vi "UHR-Fleezers Control (host) -Leonardo 04-2018 V4_fish.vi"(0 "Tab Green FB":T5(tab)=enum."Trap Control (RF)") -> ()   [LabVIEW 2014] (continued)
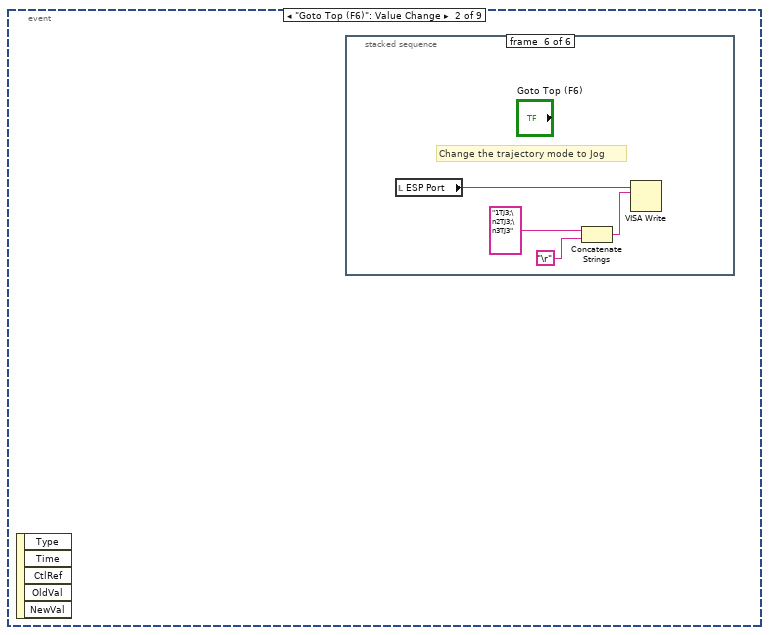
[diagram p4: hidden frame]
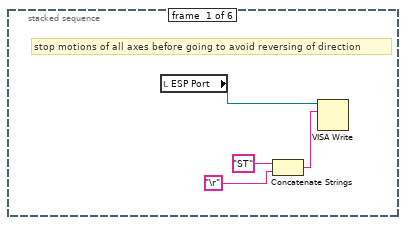
[diagram p5: hidden frame]
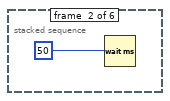
[diagram p6: hidden frame]
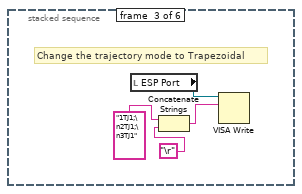
[diagram p7: hidden frame]
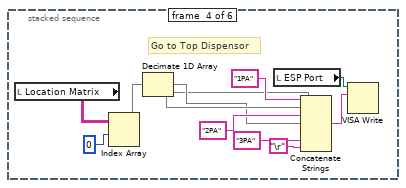
[diagram p8: hidden frame]
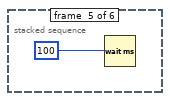
[diagram p9: hidden frame]
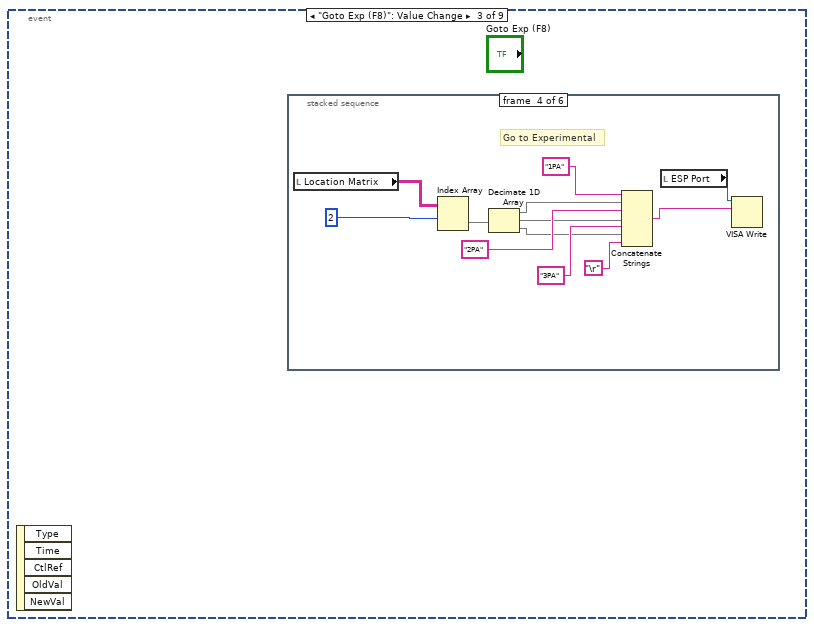
[diagram p10: hidden frame]
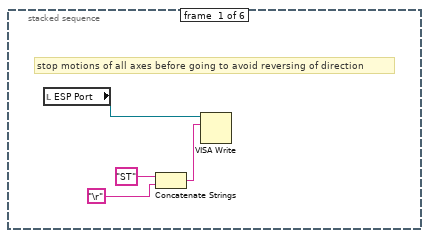
[diagram p11: hidden frame]
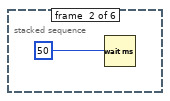
[diagram p12: hidden frame]
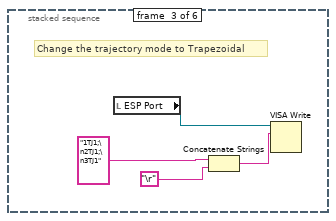
[diagram p13: hidden frame]
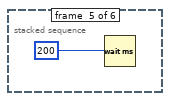
[diagram p14: hidden frame]
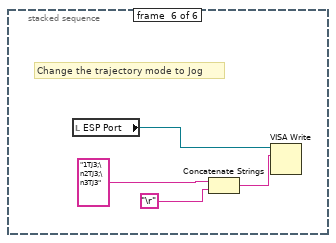
[diagram p15: hidden frame]
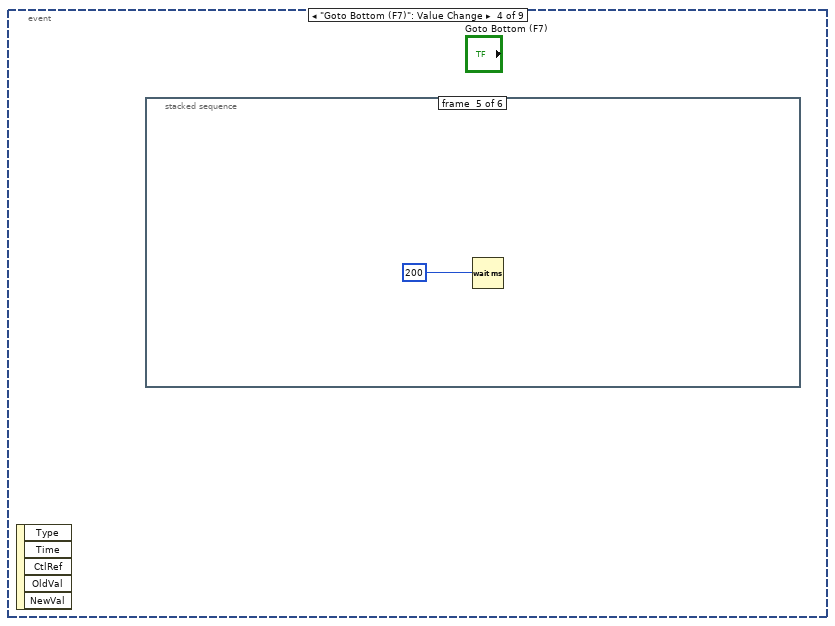
[diagram p16: hidden frame]
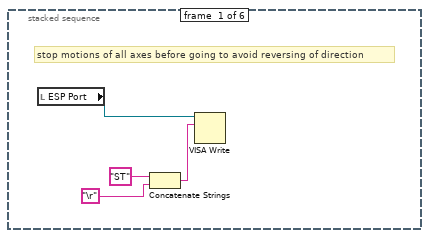
[diagram p17: hidden frame]
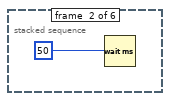
[diagram p18: hidden frame]
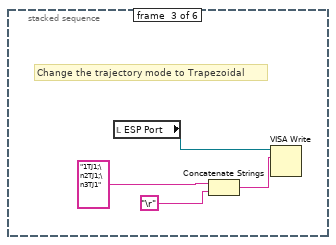
[diagram p19: hidden frame]
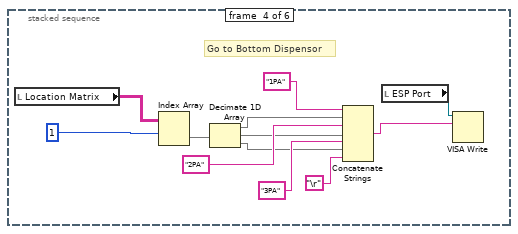
[diagram p20: hidden frame]
          tunnel: w3897 -> [_ w3916]
          tunnel: w3896 -> [_ w3915]
          tunnel: w3895 -> [_ w3913]
          tunnel: w3894 -> [_ w3911]
          tunnel: w3893 -> [_ w3910]
          tunnel: w3892 -> [_ w3909]
          tunnel: w3891 -> [_ w3908]
          tunnel: w3890 -> [_ w3907]
          tunnel: w3889 -> [_ w3906]
          tunnel: w3888 -> [_ w3905]
          frame False {
          }
          frame True {
            n2343 = Multiply(x=w3914, y=w3913) -> (x*y=→"Time (s)":dbl)
            n2344 = Less Or Equal?(x=w3914, y=w3922) -> (x <= y?=w3926:bool)
            n2345 = Or(x="Stop Saving", y="Abort save 2") -> (x .or. y?=w3918:bool)
            n2346 = Not(x=w3918) -> (.not. x?=w3927:bool)
            n2347 = And(x=w3926, y=w3927) -> (x .and. y?=w3925:bool)
            n2348 = case shown="True" w3925 {
              tunnel: w3928 -> [w3935 w4003]
              tunnel: [0.0 w4006] -> w3921
              tunnel: w3914 -> [_ w4004]
              tunnel: w3922 -> [_ w4005]
              tunnel: w3924 -> [_ w4000]
              tunnel: w3923 -> [_ _]
              tunnel: w3917 -> [w3933 w3993]
              tunnel: w3916 -> [w3932 w3994]
              tunnel: w3915 -> [_ w3992]
              tunnel: w3911 -> [_ w3991]
              tunnel: w3910 -> [_ w3945]
              tunnel: w3909 -> [_ w3984]
              tunnel: w3908 -> [_ w3962]
              tunnel: w3907 -> [w3930 w3943]
              tunnel: w3906 -> [w3931 w3942]
              tunnel: w3905 -> [_ w3939]
              frame False {
                w3929 = FALSE
                n2349 = Close File(refnum=w3935) -> ()  [unwired: 1 in, 2 out]
                n2350 = case shown="True" w3932 {
                  tunnel: w3933 -> [_ w3937]
                  frame False {
                  }
                  frame True {
                    n2351 = Close File(refnum=w3937) -> ()  [unwired: 1 in, 2 out]
                  }
                }
                n2352 = case shown="True" w3930 {
                  tunnel: w3931 -> [_ w3936]
                  frame False {
                  }
                  frame True {
                    n2353 = Close File(refnum=w3936) -> ()  [unwired: 1 in, 2 out]
                  }
                }
                n2354 = local write "Calibrating Trap..."(w3929) -> ()
                n2355 = call <vilib>:"Beep.vi"() -> ()  [unwired: 3 in, 9 out]
                n2356 = local write "Stop Saving"(w3929) -> ()
                n2357 = property on="Raster Scanning..." class="Bool (strict)"("Val(Sgnl)"=w3929) -> ()  [unwired: 2 in, 2 out]
                "Saving..." <- w3929
              }
              frame True {
                n2358 = local read "Calibrating Trap..."() -> (w3995:bool)
                n2359 = case "Write fl. data" shown="True" w3994 {
                  tunnel: w3993 -> [_ w4029]
                  tunnel: w3992 -> [_ w4028]
                  frame False {
                  }
                  frame True {
                    n2360 = Write to Binary File(file (use dialog)=w4029, data=w4028, 5:FALSE ("prepend array or string size? (T)"), 9:T30."big-endian, network order" ("byte order (0:big-endian, network order)")) -> ()  [unwired: 1 in, 4 out]
                  }
                }
                n2361 = Greater?(x="Save ave N", y=1.0) -> (0:w3998:bool)
                n2362 = Not(x=w3995) -> (.not. x?=w3997:bool)
                n2363 = And(x=w3997, y=w3998) -> (x .and. y?=w3940:bool)
                n2364 = case shown="True" w3940 {
                  tunnel: w3939 -> [w4009 w4020]
                  tunnel: [w4009 w4012] -> w3938
                  tunnel: "Save ave N" -> [_ w4013]
                  frame False {
                  }
                  frame True {
                    w4010 = 2 ("dimension size")
                    n2365 = Array Size(array=w4020) -> (size(s)=w4014:i32)
                    n2366 = Divide(x=w4014, y=w4010) -> (x/y=w4018:dbl)
                    n2367 = Reshape Array(w4020, w4018, w4010) -> (w4019:u64[][])
                    n2368 = Transpose 2D Array(2D array=w4019) -> (transposed array=w4017:u64[][])
                    n2369 = for {
                      tunnel: w4017 -> [w4022] mode=indexing
                      tunnel: [w4021] -> w4011 mode=indexing
                      tunnel: w4013 -> [w4023]
                      workers-P: _ -> [_]
                      n2370 = call "downsample 1D array - U64.vi"("Ave N"=w4023, "Array In"=w4022) -> ("Array Out"=w4021:u64[])  [unwired: 1 in]
                    }
                    n2371 = Transpose 2D Array(2D array=w4011) -> (transposed array=w4016:u64[][])
                    n2372 = Divide(x=w4014, y=w4013) -> (x/y=w4015:dbl)
                    n2373 = Reshape Array(w4016, w4015) -> (w4012:u64[])
                  }
                }
                n2374 = case shown="True" w3940 {
                  tunnel: w4000 -> [w4032 w4044]
                  tunnel: [w4032 w4036] -> w3996
                  tunnel: "Save ave N" -> [_ w4037]
                  tunnel: w3991 -> [_ w4035]
                  frame False {
                    # "don't downsample data for trap calibration"
                  }
                  frame True {
                    n2375 = Array Size(array=w4044) -> (size(s)=w4038:i32)
                    n2376 = Array Size(array=w4035) -> (size(s)=w4034:i32)
                    n2377 = Divide(x=w4038, y=w4034) -> (x/y=w4042:dbl)
                    n2378 = Reshape Array(w4044, w4042, w4034) -> (w4043:i16[][])
                    n2379 = Transpose 2D Array(2D array=w4043) -> (transposed array=w4041:i16[][])
                    n2380 = for {
                      tunnel: w4041 -> [w4047] mode=indexing
                      tunnel: [w4046] -> w4033 mode=indexing
                      tunnel: w4037 -> [w4045]
                      workers-P: _ -> [_]
                      n2381 = call "downsample 1D array - I16.vi"("Ave N"=w4045, "Array In"=w4047) -> ("Array Out"=w4046:i16[])  [unwired: 1 out]
                    }
                    n2382 = Transpose 2D Array(2D array=w4033) -> (transposed array=w4040:i16[][])
                    n2383 = Divide(x=w4038, y=w4037) -> (x/y=w4039:dbl)
                    n2384 = Reshape Array(w4040, w4039) -> (w4036:i16[])
                  }
                }
                n2385 = Index Array(array=w3962, index=1) -> (element=w3965:waveform(dbl))
                n2386 = Index Array(array=w3962, index=0) -> (element=w3967:waveform(dbl))
                n2387 = Unbundle By Name(w3965) -> ("Y"=w3969:dbl[])
                n2388 = Unbundle By Name(w3967) -> ("Y"=w3977:dbl[])
                n2389 = case "Write trap pos. data" shown="True" w3943 {
                  tunnel: w3942 -> [_ w4025]
                  tunnel: w3938 -> [_ w4024]
                  frame False {
                  }
                  frame True {
                    n2390 = Write to Binary File(file (use dialog)=w4025, data=w4024, 5:FALSE ("prepend array or string size? (T)"), 9:T30."big-endian, network order" ("byte order (0:big-endian, network order)")) -> ()  [unwired: 1 in, 4 out]
                  }
                }
                n2391 = Write to Binary File(file (use dialog)=w4003, data=w3996, 5:FALSE ("prepend array or string size? (T)"), 9:T30."big-endian, network order" ("byte order (0:big-endian, network order)")) -> ()  [unwired: 1 in, 4 out]
                n2392 = feedback #26(w3969) -> (w3971:dbl[])
                n2393 = Build Array (concatenate)(w3971, w3969) -> (w3970:dbl[])
                n2394 = Select(t=w3969, s=w3945, f=w3970) -> (s? t:f=w3955:dbl[])
                n2395 = feedback-in #26(w3955) -> ()
                n2396 = feedback #27(w3977) -> (w3990:dbl[])
                n2397 = Build Array (concatenate)(w3990, w3977) -> (w3989:dbl[])
                n2398 = Select(t=w3977, s=w3945, f=w3989) -> (s? t:f=w3964:dbl[])
                n2399 = feedback-in #27(w3964) -> ()
                n2400 = Divide(x=w4004, y=w4005) -> (x/y=w4007:dbl)
                n2401 = Multiply(x=w4007, y=100.0) -> (x*y=w4006:dbl)
                n2402 = Build Array(w3964, w3955) -> (→"Saved APD":dbl[][])
                n2403 = Array Size(array=w3964) -> (size(s)=w3982:i32)
                n2404 = Unbundle By Name(w3984) -> ("Y"=w3988:dbl[])
                n2405 = Subtract(x=w3982, y="N pts to average") -> (x-y=w3958:i32)
                n2406 = Multiply(x="N pts to average", y=u16 2) -> (x*y=w3959:u16)
                n2407 = Subtract(x=w3982, y=w3959) -> (x-y=w3957:i32)
                n2408 = feedback #28(w3988) -> (w3987:dbl[])
                n2409 = Build Array (concatenate)(w3987, w3988) -> (w3986:dbl[])
                n2410 = Select(t=w3988, s=w3945, f=w3986) -> (s? t:f=w3985:dbl[])
                "Trap Delta Graph" <- w3985
                n2411 = feedback-in #28(w3985) -> ()
                n2412 = Array Subset(array=w3964, index=w3958, length="N pts to average") -> (w3981:dbl[])
                n2413 = Array Subset(array=w3964, index=w3957, length="N pts to average") -> (w3980:dbl[])
                n2414 = Array Subset(array=w3955, index=w3958, length="N pts to average") -> (w3961:dbl[])
                n2415 = Array Subset(array=w3955, index=w3957, length="N pts to average") -> (w3960:dbl[])
                n2416 = call-poly <vilib>:"Mean.vi"("X"=w3981) -> ("mean"=w3979:dbl)  [unwired: 1 out]
                n2417 = call-poly <vilib>:"Mean.vi"("X"=w3961) -> ("mean"=w3954:dbl)  [unwired: 1 out]
                n2418 = call-poly <vilib>:"Mean.vi"("X"=w3980) -> ("mean"=w3978:dbl)  [unwired: 1 out]
                n2419 = call-poly <vilib>:"Mean.vi"("X"=w3960) -> ("mean"=w3953:dbl)  [unwired: 1 out]
                n2420 = Subtract(x=w3954, y=w3953) -> (x-y=w3944:dbl)
                "Delta Fl. 2" <- w3944
                n2421 = Subtract(x=w3979, y=w3978) -> (x-y=w3976:dbl)
                "Delta Fl. 1" <- w3976
                n2422 = Initialize Array(w3976, 1 ("dimension size")) -> (w3973:dbl[])
                n2423 = Initialize Array(w3944, 1 ("dimension size")) -> (w3950:dbl[])
                n2424 = feedback #29(w3973) -> (w3974:dbl[])
                n2425 = Build Array (concatenate)(w3974, w3973) -> (w3972:dbl[])
                n2426 = feedback #30(w3950) -> (w3951:dbl[])
                n2427 = Build Array (concatenate)(w3951, w3950) -> (w3949:dbl[])
                n2428 = Select(t=w3973, s=w3945, f=w3972) -> (s? t:f=w3948:dbl[])
                n2429 = feedback-in #29(w3948) -> ()
                n2430 = Select(t=w3950, s=w3945, f=w3949) -> (s? t:f=w3947:dbl[])
                n2431 = feedback-in #30(w3947) -> ()
                n2432 = Build Array(w3948, w3947) -> (→"Save APD Deriv":dbl[][])
              }
            }
            "Progress" <- w3921
            "Progress 2" <- w3921
          }
        }
      }
    }
    n2433 = Divide(x=w2255, y=w2256) -> (x/y=w2246:ext)
    "Trap 2 amplitude" <- w2246
    n2434 = Bundle By Name(cluster=w2508, "Green FB Ch 0"=w2507, "Green FB Ch 1"=w2506) -> (w2492:T49)
    "Green FB Signals (V)" <- w2492
    n2435 = case shown="True" w2248 {
      tunnel: w2247 -> [_ w2645]
      tunnel: w2246 -> [_ w2644]
      frame False {
      }
      frame True {
        w2646 = 50.0
        n2436 = Greater?(x=w2644, y=w2646) -> (0:w2642:bool)
        n2437 = Greater?(x=w2645, y=w2646) -> (0:w2643:bool)
        n2438 = Or(x=w2643, y=w2642) -> (x .or. y?=w2641:bool)
        n2439 = case shown="True" w2641 {
          frame False {
          }
          frame True {
            n2440 = property on="All FB On/Off" class="Bool (strict)"("Val(Sgnl)"=FALSE) -> ()  [unwired: 2 in, 2 out]
            "Feedback overload" <- TRUE
          }
        }
      }
    }
    n2441 = Unbundle By Name(w2492) -> ("Green FB Ch 2"=→"Green FB Plot":dbl)
    n2442 = local read "wait to reset values"() -> (w2576:bool)
    n2443 = Not(x=w2573) -> (.not. x?=w2577:bool)
    n2444 = And(x=w2577, y=w2576) -> (x .and. y?=w2578:bool)
    n2445 = case "Part of MCL raster scanning: returns to initial positions after scan done" shown="True" w2578 {
      tunnel: w2581 -> [w3470 w3477]
      tunnel: [w3470 w3476] -> w2580
      tunnel: w2575 -> [w3469 w3475]
      tunnel: [w3469 w3474] -> w2574
      frame False {
      }
      frame True {
        w3485 = 10.0 ("y")
        w3484 = 32767.0 ("y")
        # "to return scan values\nafter a synchronous \nAOM scan"
        n2446 = local read "AO2"() -> (w3478:dbl)
        n2447 = local read "AO1"() -> (w3479:dbl)
        n2448 = local write "wait to reset values"(FALSE ("wait to reset values")) -> ()
        n2449 = Multiply(x=w3479, y=w3484) -> (x*y=w3481:dbl)
        n2450 = Multiply(x=w3478, y=w3484) -> (x*y=w3483:dbl)
        n2451 = Divide(x=w3481, y=w3485) -> (x/y=w3480:dbl)
        n2452 = Divide(x=w3483, y=w3485) -> (x/y=w3482:dbl)
        n2453 = To Word Integer(number=w3480) -> (16bit integer=w3486:i16)
        n2454 = To Word Integer(number=w3482) -> (16bit integer=w3487:i16)
        n2455 = local read "Total Counts (ticks)"() -> (w3471:u32)
        n2456 = xnode "Read/Write Control"("FPGA VI Reference In"=w3477, "error in"=w3475, "AO1 (Y)"=w3486, "AO2 (X)"=w3487, "MCL count"=w3471) -> ("FPGA VI Reference Out"=w3476:T20, "error out"=w3474:errorcluster)
        n2457 = local read "Scan Range (V)\n(of steps)"() -> (w3472:dbl)
        n2458 = property on="Scan Range (V)\n(of steps)" class="DigNum (strict)"("Val(Sgnl)"=w3472) -> ()  [unwired: 2 in, 2 out]
      }
    }
    n2459 = node-c288() -> ()  [unwired: 2 out]
  }
  n2460 = node-c288(3 ("Processor")) -> (w109:T25)  [unwired: 3 out]
  n2461 = timed-loop "Oscillate AOD (debugging)" {
    tunnel: w62 -> [w4049]
    tunnel: [w4048] -> w73
    timing: w109 -> [_]
    timing-out: [_] -> w108
    stop <- w4048 stop-if-true
    n2462 = node-c288() -> ()  [unwired: 2 out]
    n2463 = event shown="[1] \"Fl. Triggered...\": Value Change" {
      selector: _ -> [_ _ _]
      dyn-events: _ -> [_ _ _]
      timeout: _ -> [_ _ _]
      tunnel: w4049 -> [w4056 _ _]
      tunnel: [FALSE ("Stop All") _ w4324] -> w4048
      event "Oscillate Set 2", "Fish for Tether": Value Change {
        n2464 = event-data() -> ()  [unwired: 6 out]
        n2465 = local read "Oscillate Set 2"() -> (w4055:bool)
        n2466 = Or(x=w4055, y="Fish for Tether") -> (x .or. y?=w4053:bool)
        n2467 = case shown="True" w4053 {
          tunnel: w4056 -> [_ w4059]
          tunnel: "Fish for Tether" -> [_ w4058]
          frame False {
          }
          frame True {
            n2468 = case shown="True" w4058 {
              frame False {
              }
              frame True {
                n2469 = local write "Scan axis 2"(TRUE) -> ()
                n2470 = local write "Tether"(FALSE ("Tether")) -> ()
              }
            }
            n2471 = node-c288("Period") -> (w4061:T25)  [unwired: 3 out]
            n2472 = timed-loop "Oscillate AOD" {
              timing: w4061 -> [_]
              timing-out: [_] -> w4060
              tunnel: w4059 -> [w4071]
              tunnel: w4058 -> [w4070]
              i -> [w4073]
              stop <- w4069 stop-if-true
              n2473 = node-c288() -> (w4072:i64)  [unwired: 1 out]
              n2474 = flat-sequence {
                tunnel: w4073 -> [w4099]
                tunnel: w4072 -> [w4098]
                tunnel: w4071 -> [w4082]
                tunnel: w4070 -> [w4084]
                tunnel: [w4084] -> w4068
                tunnel: [w4083] -> w4067
                tunnel: [w4081] -> w4066
                tunnel: [w4078] -> w4064
                tunnel: w4068 -> [w4135]
                tunnel: w4067 -> [w4133]
                tunnel: w4066 -> [w4132]
                tunnel: [w4131] -> w4065
                tunnel: w4064 -> [w4130]
                tunnel: [w4199] -> w4069
                tunnel: w4065 -> [w4197]
                frame #0 {
                  n2475 = Divide(x=w4098, y=i64 1000) -> (x/y=w4093:dbl)
                  n2476 = Multiply(x=w4093, y=w4099) -> (x*y=w4095:dbl)
                  n2477 = Multiply(x="Osc. freq. (Hz)", y=6.283185307179586) -> (x*y=w4096:dbl)
                  n2478 = Multiply(x=w4096, y=w4095) -> (x*y=w4080:dbl)
                  n2479 = local read "BD 1 Frequency 2 (MHz)"() -> (w4077:dbl)
                  n2480 = local read "BD 1 Frequency 1 (MHz)"() -> (w4074:dbl)
                  n2481 = case shown="True" w4084 {
                    tunnel: w4080 -> [w4105 w4112]
                    tunnel: w4077 -> [_ w4122]
                    tunnel: [w4102 w4106] -> w4085
                    tunnel: [FALSE w4115] -> w4081
                    tunnel: [0.0 w4108] -> w4078
                    tunnel: w4074 -> [_ w4107]
                    frame False {
                      n2482 = Sine(x=w4105) -> (sin(x)=w4103:dbl)
                      n2483 = Multiply(x=w4103, y="Osc. amp. (MHz)") -> (x*y=w4102:dbl)
                    }
                    frame True {
                      n2484 = Cosine(x=w4112) -> (cos(x)=w4125:dbl)
                      n2485 = Subtract(x=w4122, y=w4107) -> (x-y=w4121:dbl)
                      n2486 = Decrement(x=w4125) -> (x-1=w4124:dbl)
                      n2487 = Subtract(x=w4121, y="Closest Delta (MHz)") -> (x-y=w4118:dbl)
                      n2488 = Divide(x=w4124, y=2.0) -> (x/y=w4119:dbl)
                      n2489 = Multiply(x=w4119, y=w4118) -> (x*y=w4106:dbl)
                      n2490 = local read "Vec Mean of T1 T2"() -> (w4114:dbl[])
                      n2491 = Greater?(x=w4114, y="Stop F (pN)") -> (0:w4116:bool[])
                      n2492 = Or Array Elements(Boolean array=w4116) -> (logical OR=w4115:bool)
                      n2493 = Divide(x=w4112, y=6.283185307179586) -> (x/y=w4111:dbl)
                      n2494 = Round Toward +Infinity(x=w4111) -> (ceil(x): smallest int >= x=w4108:dbl)
                      "Attempts" <- w4108
                      n2495 = Greater?(x=w4108, y="Attempt Limit") -> (0:w4110:bool)
                      n2496 = case shown="True" w4110 {
                        frame False {
                        }
                        frame True {
                          n2497 = local write "Fish for Tether"(FALSE ("Fish for Tether")) -> ()
                          n2498 = call <vilib>:"Beep.vi"() -> ()  [unwired: 3 in, 9 out]
                          n2499 = local read "Messages"() -> (w4127:string)
                          n2500 = call "Update messages.vi"("Message to add"="Tether fishing timeout." ("Messages"), "Old message string"=w4127) -> ("New message string"=→"Messages":string)
                        }
                      }
                    }
                  }
                  n2501 = local read "Y RF Frequency Limits (MHz)"() -> (w4086:T16)
                  n2502 = local read "X RF Frequency Limits (MHz)"() -> (w4087:T16)
                  n2503 = local read "BD 1 Frequency 3 (MHz)"() -> (w4092:dbl)
                  n2504 = local read "BD 2 Frequency 2 (MHz)"() -> (w4076:dbl)
                  n2505 = Select(t=w4077, s="Scan axis 2", f=w4076) -> (s? t:f=w4088:dbl)
                  n2506 = Add(x=w4085, y=w4088) -> (x+y=w4083:dbl)
                  n2507 = Select(t=w4083, s="Scan axis 2", f=w4077) -> (s? t:f=w4075:dbl)
                  n2508 = Select(t=w4076, s="Scan axis 2", f=w4083) -> (s? t:f=w4090:dbl)
                  n2509 = local read "BD 2 Frequency 3 (MHz)"() -> (w4091:dbl)
                  n2510 = call "set RF board frequency - interlace.vi"("Board 2 Frequency Limits"=w4086, "Board 1 Frequency Limits"=w4087, "FPGA VI Reference In"=w4082, "Board 2 Frequency 3 (MHz)"=w4091, "Board 1 Frequency 3 (MHz)"=w4092, "Board 2 Frequency 2 (MHz)"=w4076, "Board 2 Frequency 1 (MHz)"=w4090, "Board 1 Frequency 2 (MHz)"=w4075, "Board 1 Frequency 1  (MHz)"=w4074) -> ()  [unwired: 1 in, 2 out]
                }
                frame #1 {
                  n2511 = And(x=w4135, y=w4132) -> (x .and. y?=w4134:bool)
                  n2512 = case "Only if were fishing and now formed tether" shown="True" w4134 {
                    tunnel: w4133 -> [w4137 w4149]
                    tunnel: [w4136 w4148] -> w4131
                    tunnel: w4130 -> [_ w4144]
                    frame False {
                      n2513 = local read "Fish for Tether"() -> (w4136:bool)
                      n2514 = case shown="True" w4136 {
                        tunnel: w4137 -> [_ _]
                        frame False {
                        }
                        frame True {
                        }
                      }
                    }
                    frame True {
                      w4148 = FALSE ("Fish for Tether")
                      n2515 = call <vilib>:"Beep.vi"() -> ()  [unwired: 3 in, 9 out]
                      n2516 = Number To Decimal String(number=w4144, width (-)=i16 1) -> (decimal integer string=w4142:string)
                      n2517 = case shown="\"2\", \"3\", \"4\", \"5\", \"6\"" "Then..." {
                        selector: "Then..." -> [_ w4152]
                        tunnel: w4149 -> [w4151 _]
                        frame "1", Default {
                          # "do nothing"
                          n2518 = property on="BD 1 Frequency 1 (MHz)" class="DigNum (strict)"("Val(Sgnl)"=w4151) -> ()  [unwired: 2 in, 2 out]
                        }
                        frame "2", "3", "4", "5", "6" {
                          n2519 = flat-sequence {
                            tunnel: w4152 -> [w4154]
                            frame #0 {
                              n2520 = property on="Trap Delta (MHz)" class="DigNum (strict)"("Val(Sgnl)"="Move to Delta 1 (MHz)") -> ()  [unwired: 2 in, 2 out]
                            }
                            frame #1 {
                              n2521 = case shown="\"5\", \"6\"" w4154 {
                                selector: w4154 -> [w4157 w4167 _]
                                frame "3", "4" {
                                n2522 = flat-sequence {
                                tunnel: w4157 -> [w4158]
                                tunnel: [w4158] -> w4155
                                tunnel: [w4160] -> w4156
                                tunnel: w4155 -> [w4160]
                                tunnel: w4156 -> [w4164]
                                frame #0 {
                                n2523 = property on="Green Laser ON/Interlacing" class="Bool (strict)"("Val(Sgnl)"=TRUE ("Value (Signaling)")) -> ()  [unwired: 2 in, 2 out]
                                }
                                frame #1 {
                                n2524 = Multiply(x="Wait Before Save (s)", y=u32 1000 ("x")) -> (x*y=w4162:u32)
                                n2525 = Wait (ms)(milliseconds to wait=w4162) -> ()  [unwired: 1 out]
                                }
                                frame #2 {
                                n2526 = property on="Start Saving" class="Bool (strict)"("Value"=TRUE ("Start Saving")) -> ()  [unwired: 2 in, 2 out]
                                n2527 = case shown="Default" w4164 {
                                frame Default {
                                }
                                frame "4" {
                                n2528 = property on="Fl. Triggered..." class="Bool (strict)"("Val(Sgnl)"=TRUE ("Value (Signaling)")) -> ()  [unwired: 2 in, 2 out]
                                }
                                }
                                }
                                }
                                }
                                frame "5", "6" {
                                n2529 = stacked-sequence {
                                tunnel: w4167 -> [_ _ _ _ _ _ _ _ w4184 _ _]
                                frame #0 {
                                n2530 = Replace Array Subset(array=u32[] [0] ("Index Values"), new element="Raster Set Upon Tether", index=0) -> (w4168:u32[])
                                n2531 = property on="Saved AOD Raster Scan Parameter Sets" class="Arr (strict)"("Index Values"=w4168) -> ()  [unwired: 2 in, 2 out]
                                }
                                frame #1 {
                                n2532 = Wait (ms)(milliseconds to wait=u32 500) -> ()  [unwired: 1 out]
                                }
                                frame #2 {
                                n2533 = property on="Load parameters" class="Bool (strict)"("Val(Sgnl)"=TRUE ("Value (Signaling)")) -> ()  [unwired: 2 in, 2 out]
                                }
                                frame #3 {
                                n2534 = Wait (ms)(milliseconds to wait=u32 500) -> ()  [unwired: 1 out]
                                }
                                frame #4 {
                                n2535 = property on="Trap Raster Scan" class="Bool (strict)"("Val(Sgnl)"=TRUE ("Value (Signaling)")) -> ()  [unwired: 2 in, 2 out]
                                }
                                frame #5 {
                                n2536 = Wait (ms)(milliseconds to wait=u32 2000) -> ()  [unwired: 1 out]
                                }
                                frame #6 {
                                n2537 = while {
                                stop <- w4179 stop-if-true
                                n2538 = local read "Raster Scanning..."() -> (w4178:bool)
                                n2539 = local read "Saving..."() -> (w4181:bool)
                                n2540 = Wait (ms)(milliseconds to wait=u32 100) -> ()  [unwired: 1 out]
                                n2541 = Not(x=w4181) -> (.not. x?=w4180:bool)
                                n2542 = Not(x=w4178) -> (.not. x?=w4177:bool)
                                n2543 = And(x=w4180, y=w4177) -> (x .and. y?=w4179:bool)
                                }
                                }
                                frame #7 {
                                n2544 = property on="Trap Delta (MHz)" class="DigNum (strict)"("Val(Sgnl)"="Move to Delta 2 (MHz)") -> ()  [unwired: 2 in, 2 out]
                                }
                                frame #8 {
                                n2545 = local read "Tether"() -> (w4185:bool)
                                n2546 = case shown="True" w4185 {
                                tunnel: w4184 -> [_ w4186]
                                frame False {
                                }
                                frame True {
                                n2547 = flat-sequence {
                                tunnel: w4186 -> [w4188]
                                frame #0 {
                                n2548 = Wait (ms)(milliseconds to wait=u32 500) -> ()  [unwired: 1 out]
                                }
                                frame #1 {
                                n2549 = case shown="\"6\"" w4188 {
                                frame Default {
                                }
                                frame "6" {
                                n2550 = property on="Green Laser ON/Interlacing" class="Bool (strict)"("Val(Sgnl)"=TRUE ("Green Laser ON/Interlacing")) -> ()  [unwired: 2 in, 2 out]
                                }
                                }
                                }
                                frame #2 {
                                n2551 = Wait (ms)(milliseconds to wait=u32 500) -> ()  [unwired: 1 out]
                                }
                                frame #3 {
                                n2552 = local write "Start Saving"("Save at end (5, 6)") -> ()
                                }
                                }
                                }
                                }
                                }
                                frame #9 {
                                n2553 = local read "Bead Sep. Int. Time (s)"() -> (w4194:dbl)
                                n2554 = Multiply(x=w4194, y=1000.0) -> (x*y=w4193:dbl)
                                n2555 = Wait (ms)(milliseconds to wait=w4193) -> ()  [unwired: 1 out]
                                }
                                frame #10 {
                                n2556 = property on="Rescale on Mean" class="Bool (strict)"("Val(Sgnl)"=TRUE ("Value (Signaling)")) -> ()  [unwired: 2 in, 2 out]
                                }
                                }
                                }
                                frame "2", Default {
                                }
                              }
                            }
                          }
                        }
                      }
                      n2557 = Concatenate Strings("Formed tether in ", w4142, " attempt(s)." ("string")) -> (w4139:string)
                      n2558 = local read "Messages"() -> (w4146:string)
                      n2559 = local write "Fish for Tether"(w4148) -> ()
                      n2560 = call "Update messages.vi"("Message to add"=w4139, "Old message string"=w4146) -> ("New message string"=w4145:string)
                      n2561 = local write "Messages"(w4145) -> ()
                      n2562 = Get Date/Time In Seconds() -> (seconds since 1Jan1904=→"Time tether formed":timestamp)
                      "Tether" <- "Tether Alarm?"
                    }
                  }
                }
                frame #2 {
                  n2563 = local read "Oscillate Set 2"() -> (w4198:bool)
                  n2564 = local read "Stop All"() -> (w4200:bool)
                  n2565 = Not Or(1:w4197, 2:w4198) -> (0:w4196:bool)
                  n2566 = Compound Arithmetic op=OR(w4200, w4196) -> (w4199:bool)
                }
              }
              n2567 = node-c288() -> ()  [unwired: 2 out]
            }
            n2568 = node-c288(w4060) -> ()  [unwired: 1 out]
          }
        }
      }
      event "Fl. Triggered...": Value Change {
        n2569 = event-data() -> ()  [unwired: 7 out]
        n2570 = case shown="True" "Fl. Triggered..." {
          frame False {
          }
          frame True {
            n2571 = node-c288() -> (w4212:T25)  [unwired: 4 out]
            n2572 = timed-loop {
              timing: w4212 -> [_]
              timing-out: [_] -> w4211
              tunnel: "Action" -> [w4216]
              shift-right: [w4213] -> _
              shift-left: u8 255 -> [w4215]
              stop <- w4217 stop-if-true
              n2573 = node-c288() -> ()  [unwired: 2 out]
              n2574 = flat-sequence {
                tunnel: w4216 -> [w4229]
                tunnel: w4215 -> [w4226]
                tunnel: [w4225] -> w4214
                tunnel: [w4315] -> w4217
                tunnel: w4214 -> [w4314]
                tunnel: [w4314] -> w4213
                frame #0 {
                  n2575 = local read "Delta Fl. 2"() -> (w4220:dbl)
                  n2576 = local read "Delta Fl. 1"() -> (w4221:dbl)
                  n2577 = Select(t=w4221, s="APD to Watch", f=w4220) -> (s? t:f=w4219:dbl)
                  n2578 = Multiply(x="Fl. Delta Thresh. (kHz)", y=1000.0) -> (x*y=w4228:dbl)
                  n2579 = Greater?(x=w4219, y=w4228) -> (0:w4223:bool)
                  n2580 = Or(x="Force Yank", y=w4223) -> (x .or. y?=w4224:bool)
                  n2581 = case shown="True" w4224 {
                    tunnel: w4229 -> [_ w4239]
                    tunnel: w4226 -> [w4231 w4235]
                    tunnel: [w4231 w4232] -> w4225
                    frame False {
                    }
                    frame True {
                      n2582 = flat-sequence {
                        tunnel: w4236 -> [w4245]
                        tunnel: [w4245] -> w4240
                        tunnel: w4239 -> [w4244]
                        tunnel: [w4244] -> w4238
                        tunnel: [w4243] -> w4237
                        tunnel: w4235 -> [w4242]
                        tunnel: [w4241] -> w4234
                        tunnel: w4240 -> [w4270]
                        tunnel: w4238 -> [w4269]
                        tunnel: w4237 -> [w4268]
                        tunnel: w4234 -> [w4267]
                        tunnel: [w4267] -> w4233
                        tunnel: w4233 -> [w4312]
                        tunnel: [w4312] -> w4232
                        frame #0 {
                          n2583 = call <vilib>:"Beep.vi"() -> ()  [unwired: 3 in, 9 out]
                          n2584 = local write "Waiting"(FALSE ("Waiting")) -> ()
                          n2585 = Increment(x=w4242) -> (x+1=w4241:u8)
                          n2586 = case shown="\"Yank\"" w4244 {
                            tunnel: w4241 -> [_ _ w4251]
                            frame "Image" {
                              n2587 = property on="Confocal Image" class="Bool (strict)"("Val(Sgnl)"=TRUE ("Value (Signaling)")) -> ()  [unwired: 2 in, 2 out]
                            }
                            frame "Alarm", Default {
                            }
                            frame "Yank" {
                              n2588 = flat-sequence {
                                tunnel: w4251 -> [w4254]
                                tunnel: [w4253] -> w4250
                                tunnel: ["N Array El"] -> w4249
                                tunnel: w4250 -> [w4264]
                                tunnel: w4249 -> [w4260]
                                frame #0 {
                                n2589 = Multiply(x="Yank Delay (s)", y=1000.0) -> (x*y=w4257:dbl)
                                n2590 = Quotient & Remainder(x=w4254, y="N Array El") -> (x-y*floor(x/y)=w4253:u8)  [unwired: 1 out]
                                n2591 = Wait (ms)(milliseconds to wait=w4257) -> ()  [unwired: 1 out]
                                }
                                frame #1 {
                                n2592 = Random Number (0-1)() -> (number: 0 to 1=w4261:dbl)
                                n2593 = Multiply(x=w4260, y=w4261) -> (x*y=w4259:dbl)
                                n2594 = Round Toward -Infinity(1:w4259) -> (0:w4258:dbl)
                                n2595 = Select(t=w4258, s="Random Choice", f=w4264) -> (s? t:f=w4262:dbl)
                                n2596 = Index Array(array="Yank to Delta Array (MHz)", index=w4262) -> (element=w4265:dbl)
                                n2597 = property on="Trap Delta (MHz)" class="DigNum (strict)"("Val(Sgnl)"=w4265) -> ()  [unwired: 2 in, 2 out]
                                }
                              }
                            }
                          }
                          n2598 = local read "Time (s)"() -> (w4243:dbl)
                          "Fl. High" <- TRUE ("Yanking")
                        }
                        frame #1 {
                          n2599 = node-c288() -> (w4272:T25)  [unwired: 4 out]
                          n2600 = timed-loop {
                            timing: w4272 -> [_]
                            timing-out: [_] -> w4271
                            tunnel: w4270 -> [w4288]
                            tunnel: w4269 -> [w4286]
                            tunnel: w4268 -> [w4285]
                            stop <- w4287 stop-if-true
                            n2601 = node-c288() -> ()  [unwired: 2 out]
                            n2602 = local read "Fl. Delta Thresh. (kHz)"() -> (w4280:dbl)
                            n2603 = local read "Fl. Triggered..."() -> (w4289:bool)
                            n2604 = local read "Delta Fl. 1"() -> (w4276:dbl)
                            n2605 = local read "Delta Fl. 2"() -> (w4274:dbl)
                            n2606 = local read "Stop All"() -> (w4283:bool)
                            n2607 = local read "APD to Watch"() -> (w4275:bool)
                            n2608 = Select(t=w4276, s=w4275, f=w4274) -> (s? t:f=w4273:dbl)
                            n2609 = Not(x=w4289) -> (.not. x?=w4284:bool)
                            n2610 = Multiply(x=w4280, y=1000.0) -> (x*y=w4279:dbl)
                            n2611 = Negate(x=w4279) -> (-x=w4278:dbl)
                            n2612 = Less?(x=w4273, y=w4278) -> (x < y?=w4282:bool)
                            n2613 = Compound Arithmetic op=OR(w4282, w4283, w4284, "Force Reset") -> (w4287:bool)
                            n2614 = case shown="True" w4287 {
                              tunnel: w4288 -> [_ w4300]
                              tunnel: w4286 -> [_ w4299]
                              tunnel: w4285 -> [_ w4297]
                              frame False {
                              }
                              frame True {
                                n2615 = case shown="\"Yank\"" w4299 {
                                tunnel: w4300 -> [_ w4301]
                                frame "Image", Default {
                                }
                                frame "Yank" {
                                n2616 = flat-sequence {
                                tunnel: [w4306] -> w4302
                                tunnel: w4301 -> [w4306]
                                tunnel: w4302 -> [w4307]
                                frame #0 {
                                n2617 = local read "Yank Delay (s)"() -> (w4305:dbl)
                                n2618 = Multiply(x=w4305, y=1000.0) -> (x*y=w4303:dbl)
                                n2619 = Wait (ms)(milliseconds to wait=w4303) -> ()  [unwired: 1 out]
                                }
                                frame #1 {
                                n2620 = property on="Trap Delta (MHz)" class="DigNum (strict)"("Val(Sgnl)"=w4307) -> ()  [unwired: 2 in, 2 out]
                                }
                                }
                                }
                                }
                                n2621 = local read "Time (s)"() -> (w4298:dbl)
                                n2622 = Subtract(x=w4298, y=w4297) -> (x-y=w4294:dbl)
                                "Duration (s)" <- w4294
                                n2623 = Number To Decimal String(number=w4294, width (-)=i16 0) -> (decimal integer string=w4292:string)
                                n2624 = Concatenate Strings(w4292, " s fluorescence event." ("string")) -> (w4290:string)
                                n2625 = local read "Messages"() -> (w4296:string)
                                n2626 = call "Update messages.vi"("Message to add"=w4290, "Old message string"=w4296) -> ("New message string"=w4295:string)
                                n2627 = call <vilib>:"Beep.vi"() -> ()  [unwired: 3 in, 9 out]
                                n2628 = local write "Messages"(w4295) -> ()
                              }
                            }
                            n2629 = node-c288() -> ()  [unwired: 2 out]
                          }
                          n2630 = node-c288(w4271) -> ()  [unwired: 1 out]
                        }
                        frame #2 {
                          n2631 = local write "Fl. High"(FALSE ("Yanking")) -> ()
                        }
                      }
                      n2632 = local read "Trap Delta (MHz)"() -> (w4236:dbl)
                    }
                  }
                }
                frame #1 {
                  n2633 = local read "Stop All"() -> (w4318:bool)
                  n2634 = local read "Fl. Triggered..."() -> (w4316:bool)
                  n2635 = Not(x=w4316) -> (.not. x?=w4317:bool)
                  n2636 = Or(x=w4317, y=w4318) -> (x .or. y?=w4315:bool)
                  n2637 = Not(x=w4315) -> (.not. x?=→"Waiting":bool)
                }
              }
              n2638 = node-c288() -> ()  [unwired: 2 out]
            }
            n2639 = node-c288(w4211) -> ()  [unwired: 1 out]
          }
        }
      }
      event "Stop All": Value Change {
        n2640 = event-data() -> ()  [unwired: 7 out]
        n2641 = local read "Stop All"() -> (w4324:bool)
      }
    }
    n2642 = node-c288() -> ()  [unwired: 2 out]
  }
  n2643 = node-c288(w108) -> ()  [unwired: 1 out]
  n2644 = node-c288(w195) -> ()  [unwired: 1 out]
  n2645 = flat-sequence "@Alex - Set stage to 0,0,0 on exit" {
    tunnel: w3 -> [w4326]
    tunnel: [w4325] -> w2
    frame #0 {
      n2646 = local read "ESP Port"() -> (w4330:refnum<visa-resource-name>)
      n2647 = Concatenate Strings("1PA0;\n2PA0;\n3PA0" ("write buffer"), "\r") -> (w4327:string)
      n2648 = VISA Write(VISA resource name=w4330, write buffer=w4327, error in (no error)=w4326) -> (error out=w4325:errorcluster)  [unwired: 2 out]
    }
  }
  n2649 = flat-sequence {
    tunnel: w70 -> [w4335]
    tunnel: [w4334] -> w76
    tunnel: [w4331] -> w75
    tunnel: w74 -> [_]
    tunnel: w73 -> [_]
    tunnel: w72 -> [_]
    tunnel: w71 -> [_]
    tunnel: w2 -> [w4332]
    tunnel: w76 -> [w4338]
    tunnel: w75 -> [w4337]
    frame #0 {
      w4333 = FALSE ("APD to FIFO")
      n2650 = xnode "Read/Write Control"("FPGA VI Reference In"=w4335, "error in"=w4332, "APD to FIFO"=w4333, "AI to FIFO"=w4333) -> ("FPGA VI Reference Out"=w4334:T20, "error out"=w4331:errorcluster)
    }
    frame #1 {
      n2651 = xnode "Invoke Method"("FPGA VI Reference In"=w4338, "error in"=w4337) -> ("FPGA VI Reference Out"=w4336:T20)  [unwired: 1 out]
      n2652 = xnode "Close FPGA VI Reference"("FPGA VI Reference In"=w4336) -> ()  [unwired: 1 in, 1 out]
    }
  }
  "Fish Status" <- w1
